vi "String to Flags.vi"(9 "length":i32, 10 "offset":i32, 11 "string":string) -> (3 "flags":T1)   [LabVIEW 2017, in "GW Instek PSP-405.lvlib"]
doc: "Converts <b>string</b> command response into a boolean flags."
uses:
  GW Instek PSP-405.lvlib
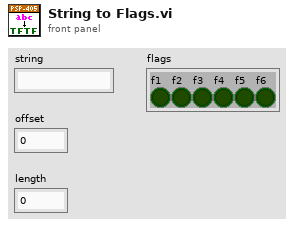
[diagram p1: front panel]
types:
  T1 = cluster{"f1":bool, "f2":bool, "f3":bool, "f4":bool, "f5":bool, "f6":bool}
  T2 = cluster{"[0]":bool, "[1]":bool, "[2]":bool, "[3]":bool, "[4]":bool, "[5]":bool}
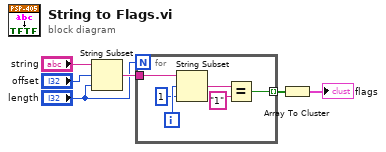
[diagram p0: block diagram]
diagram:
  n1 = String Subset(string="string", offset (0)="offset", length (rest)="length") -> (substring=w5:string)
  n2 = for {
    N: "length" -> [_]
    tunnel: w5 -> [w12]
    tunnel: [w7] -> w6 mode=indexing
    i -> [w11]
    n3 = String Subset(string=w12, offset (0)=w11, length (rest)=1 ("length (rest)")) -> (substring=w9:string)
    n4 = Equal?(x=w9, y="1") -> (x = y?=w7:bool)
  }
  n5 = Array To Cluster(array=w6) -> (cluster=→"flags":T2)
